vi "Get Keep Clean Time.vi"(11 "KeepCleanTime":sgl) -> (2 "function return":u32, 3 "KeepCleanTime out":sgl)   [LabVIEW 2018, in "AndorSDK.lvlib"]
doc: "EXPNETTYPE unsigned int WINAPI GetKeepCleanTime(float * KeepCleanTime);"
uses:
  AndorSDK.lvlib
  ATMCD32D.dll
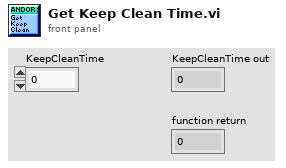
[diagram p1: front panel]
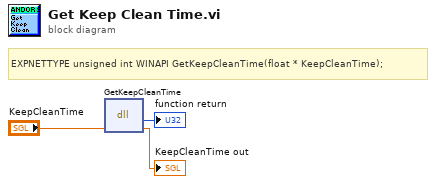
[diagram p0: block diagram]
diagram:
  # "EXPNETTYPE unsigned int WINAPI GetKeepCleanTime(float * KeepCleanTime);"
  n1 = dll-call lib="PTH2babs E\nPersönliches02 - Arbeit03-HiwijobsLabviewCodelibANDOR\tAndor SDK\nATMCD32D.*" fn="GetKeepCleanTime"("KeepCleanTime"="KeepCleanTime") -> (→"function return":u32, "KeepCleanTime"=→"KeepCleanTime out":sgl)  [unwired: 3 in, 2 out]
